vi "ICM Simple Read Program(NoScaling).vi"() -> ()   [LabVIEW 2024]
doc: "Test Program.vi\n\nThis is a simple program that uses the ICM to demonstrate its structure.\n\nInstrument Communication Module Version 1.0\nDecember, 2017 Original Code Consulting David Thomson\n www.originalcode.com"
uses:
  Query/Query.lvclass/Query.ctl
  Query/Read Cycle Time (ms).vi
  Initialize/Initialize.lvclass
  Parser/Parser.lvclass
  Query/Query.lvclass
  Bus/Bus.lvclass
panel:
  in  "stop":bool
  out "Enabled Channels":string[](array[string])
  out "Data Values":dbl[](array[numeric])
  out "String Read":string
  out "error out":errorcluster
  out "Config File":path
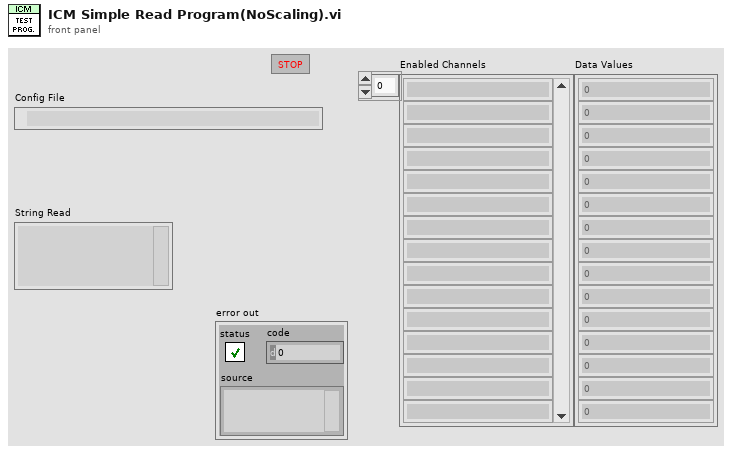
[diagram p1: front panel]
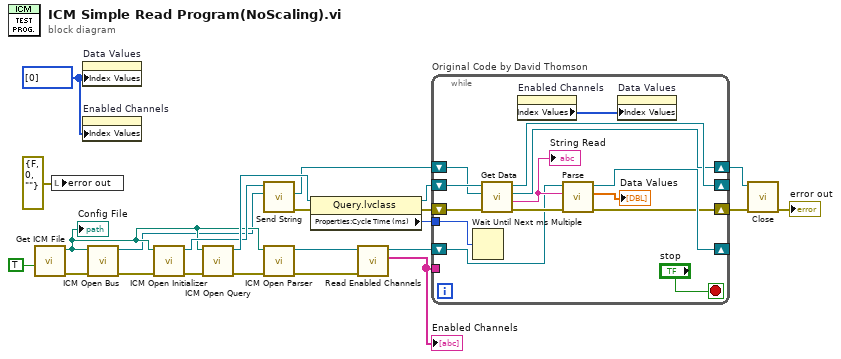
[diagram p0: block diagram]
diagram:
  w3 = u32[] [0] ("Index Values")
  n1 = call "Get ICM File.vi"("Re-Init?"=TRUE) -> ("error out"=w16:errorcluster, "ICM File"=w5:path)  [unwired: 9 in]
  "Config File" <- w5
  n2 = local write "error out"(errorcluster {"status"=FALSE, "code"=0, "source"=""} ("error out")) -> ()
  n3 = property on="Data Values" class="Arr (strict)"("Index Values"=w3) -> ()  [unwired: 2 in, 2 out]
  n4 = property on="Enabled Channels" class="Arr (strict)"("Index Values"=w3) -> ()  [unwired: 2 in, 2 out]
  n5 = call "ICM Open Bus.vi"("error in (no error)"=w16, "ICM File In"=w5) -> ("error out"=w8:errorcluster, "Bus out"=w1:refnum<class "Bus.lvclass">)  [unwired: 8 in]
  n6 = call "ICM Open Initializer.vi"("error in (no error)"=w8, "ICM File In"=w5) -> ("error out"=w4:errorcluster, "Init out"=w7:refnum<class "Initialize.lvclass">)  [unwired: 8 in]
  n7 = call "ICM Open Query.vi"("error in (no error)"=w4, "ICM File In"=w5) -> ("error out"=w17:errorcluster, "Query out"=w14:refnum<class "Query.lvclass">)  [unwired: 8 in]
  n8 = call-dynamic "Send String.vi"("Bus In"=w1, "Init in"=w7) -> ("error out"=w6:errorcluster, "Bus Out"=w2:refnum<class "Bus.lvclass">)  [unwired: 5 in, 1 out]
  n9 = call "ICM Open Parser.vi"("error in (no error)"=w17, "ICM File In"=w5) -> ("error out"=w18:errorcluster, "Parser out"=w19:refnum<class "Parser.lvclass">)  [unwired: 8 in]
  n10 = property class="Query.lvclass"(reference=w14, error in=w6) -> (reference out=w13:refnum<class "Query.lvclass">, error out=w11:errorcluster, "Properties:Cycle Time (ms)"=w12:u32)
  n11 = call-dynamic "Read Enabled Channels.vi"("error in (no error)"=w18, "Parser in"=w19) -> ("Enabled Channels"=w15:string[], "Parser out"=w9:refnum<class "Parser.lvclass">)  [unwired: 7 in, 1 out]
  "Enabled Channels" <- w15
  n12 = while "Original Code by David Thomson" {
    shift-right: [w24] -> w21
    shift-left: w11 -> [w35]
    tunnel: w12 -> [w33]
    tunnel: w15 -> [_]
    shift-right: [w25] -> w22
    shift-left: w2 -> [w32]
    shift-right: [w29] -> _
    shift-left: w9 -> [w30]
    shift-right: [w28] -> _
    shift-left: w13 -> [w36]
    stop <- "stop" stop-if-true
    n13 = Wait Until Next ms Multiple(millisecond multiple=w33) -> ()  [unwired: 1 out]
    n14 = call-dynamic "Get Data.vi"("error in (no error)"=w35, "Bus In"=w32, "Query in"=w36) -> ("error out"=w34:errorcluster, "String Read"=w37:string, "Bus Out"=w25:refnum<class "Bus.lvclass">, "Query out"=w28:refnum<class "Query.lvclass">)  [unwired: 5 in]
    "String Read" <- w37
    n15 = property on="Enabled Channels" class="Arr (strict)"() -> ("Index Values"=w27:u32[])  [unwired: 2 in, 2 out]
    n16 = call-dynamic "Parse.vi"("error in (no error)"=w34, "Data String"=w37, "Parser in"=w30) -> ("error out"=w24:errorcluster, "Data Values"=→"Data Values":dbl[], "Parser out"=w29:refnum<class "Parser.lvclass">)  [unwired: 6 in]
    n17 = property on="Data Values" class="Arr (strict)"("Index Values"=w27) -> ()  [unwired: 2 in, 2 out]
  }
  n18 = call-dynamic "Close.vi"("error in (no error)"=w21, "Bus in"=w22) -> ("error out"=→"error out":errorcluster)  [unwired: 8 in, 1 out]
